vi "Generate Event XML.vi"(11 "Events":T1[](array[typedef])) -> (3 "Event XML":string)   [LabVIEW 2015, in "NI_AWS_S3.lvlib"]
uses:
  NI_AWS_S3.lvlib
  Event.ctl
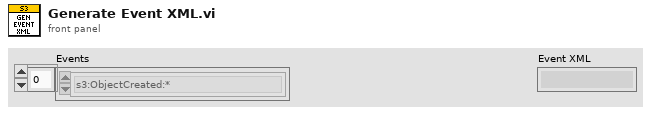
[diagram p1: front panel]
types:
  T1 = typedef "NI_AWS_S3.lvlib/Event.ctl" = enum16{"s3:ObjectCreated:*", "s3:ObjectCreated:Put", "s3:ObjectCreated:Post", "s3:ObjectCreated:Copy", "s3:ObjectCreated:CompleteMultipartUpload", "s3:ObjectRemoved:*", "s3:ObjectRemoved:Delete", "s3:ObjectRemoved:DeleteMarkerCreated", "s3:ReducedRedundancyLostObject"}
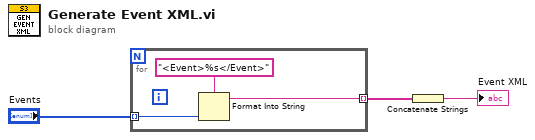
[diagram p0: block diagram]
diagram:
  n1 = for {
    tunnel: "Events" -> [w5] mode=indexing
    tunnel: [w6] -> w3 mode=indexing
    n2 = Format Into String(format string="<Event>%s</Event>", w5) -> (resulting string=w6:string)  [unwired: 2 in, 1 out]
  }
  n3 = Concatenate Strings(w3) -> (→"Event XML":string)
